vi "Modbus Slave Write Time.vi"() -> ()   [LabVIEW 2021]
doc: "An example of the modbus master functionality."
uses:
  Modbus_v121c/Network Protocol/Network Slave/daemon status.ctl
  Modbus_v121c/Network Protocol/Network Slave/TCP/Connection.ctl
  Modbus_v121c/Data Model/Identification Parameters.ctl
  Modbus_v121c/API/Slave/Modbus Slave.lvclass
  Modbus_v121c/Data Model/Device Data Model.lvclass
  Modbus_v121c/API/Wrapper/API Main.lvlib
  Modbus_v121c/Network Protocol/Network Slave/Network Slave.lvclass
  Modbus_v121c/Network Protocol/Network Slave/TCP/TCP Slave.lvclass
panel:
  out "TCP Connection List":T1[](array[typedef])=[{"Connected?"=TRUE, "IP address"="127.0.0.1", "connection error"={"status"=FALSE, "code"=0, "source"=""}}]
  out "TCP Connection Count":u32
  out "Daemon Error":errorcluster
  out "Daemon Status":T2
  in  "Port":u16=502
  in  "Basic Objects":string[](array[string])=["National Instruments", "42", "1.0.0"]
  out "Status":string
  out "Holding Registers":u16[](array[numeric])
  in  "Input Registers":u16[](array[numeric])=[0, 0, 0, 0, 0, 0, 0, 0]
  out "Coils":bool[](array[boolean])
  in  "Discrete Inputs":bool[](array[boolean])
  # "Holding Registers are the integer outputs of a modbus device. This example allows you to read the first 8 outputs."
  # "Coils are the boolean outputs of a modbus device. This example allows you to read the first 8 outputs."
  # "Modbus devices can also store objects in their memory, which are variable length strings. This example sets the basic level of objects."
  # "Discrete inputs are the boolean inputs of a modbus device. This example allows you to set the first 8 inputs."
  # "Input Registers are the integer inputs of a modbus device. This example allows you to set the first 8 inputs."
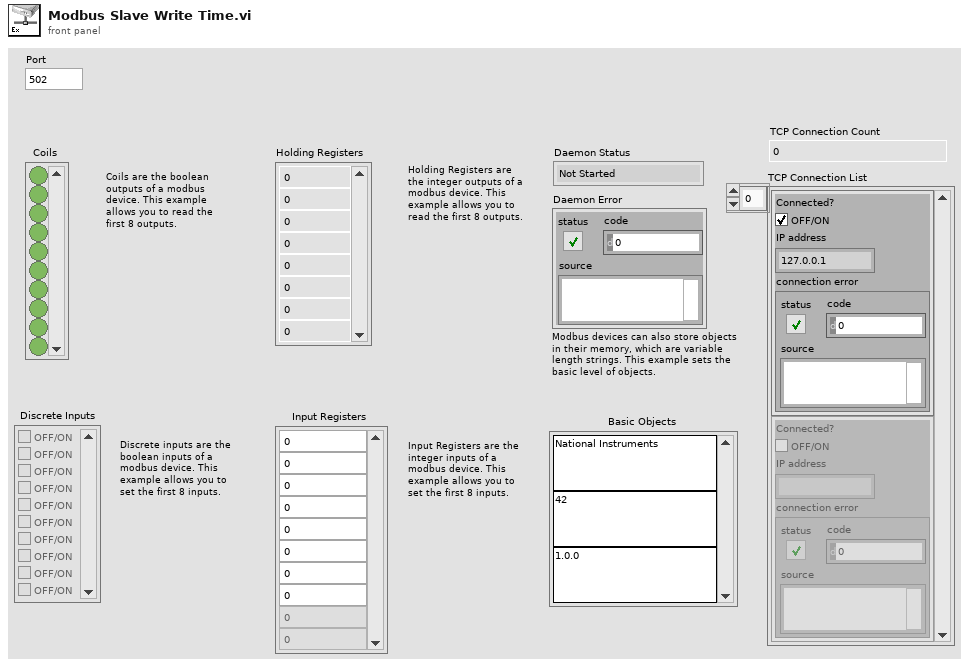
[diagram p1: front panel]
types:
  T1 = typedef "TCP Slave.lvclass/Connection.ctl" = cluster{"Connected?":bool, "IP address":string, "connection error":errorcluster}
  T2 = typedef "Network Slave.lvclass/daemon status.ctl" = enum16{"Not Started", "Running", "Error", "Stopped"}
  T3 = typedef "Device Data Model.lvclass/Identification Parameters.ctl" = cluster{"Object ID":u8, "Value":string}
  T4 = enum16{"Not Started", "Running", "Error", "Stopped"}
  T5 = cluster{"Connected?":bool, "IP address":string, "connection error":errorcluster}[]
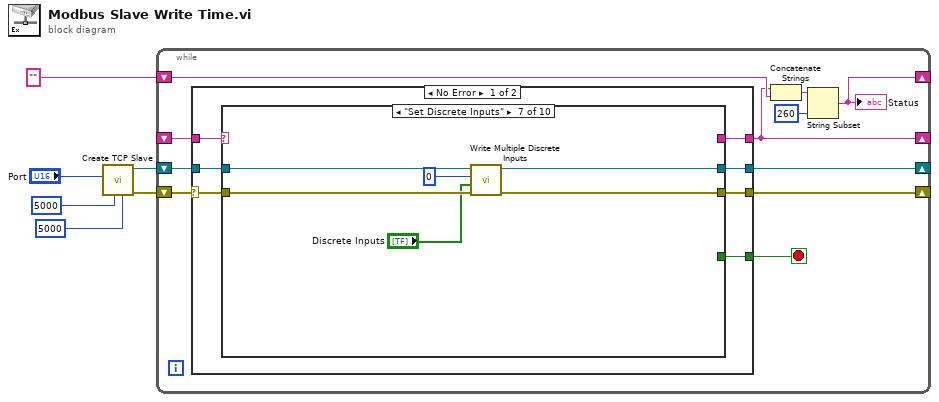
[diagram p0: block diagram]
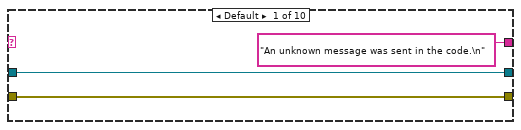
[diagram p2: hidden frame]
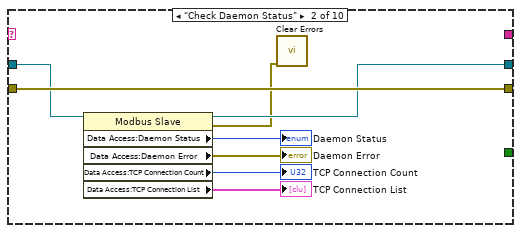
[diagram p3: hidden frame]
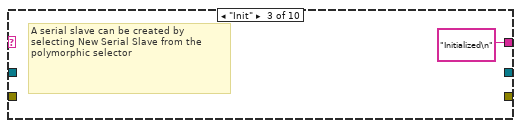
[diagram p4: hidden frame]
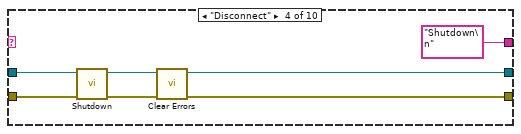
[diagram p5: hidden frame]
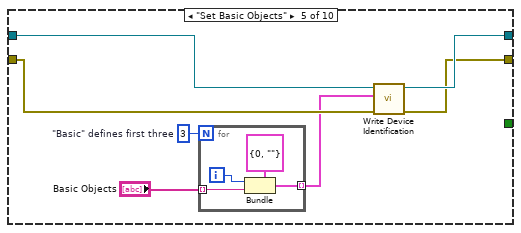
[diagram p6: hidden frame]
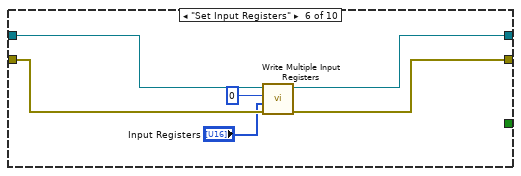
[diagram p7: hidden frame]
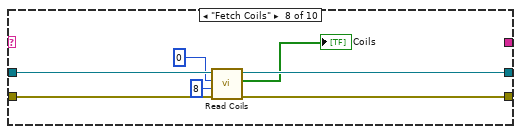
[diagram p8: hidden frame]
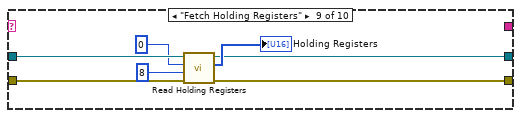
[diagram p9: hidden frame]
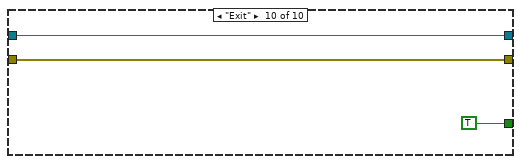
[diagram p10: hidden frame]
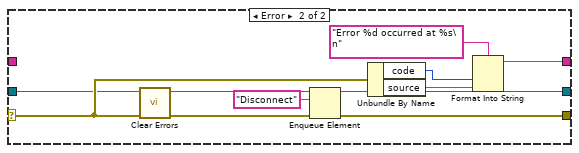
[diagram p11: hidden frame]
diagram:
  n1 = call "Create TCP Slave.vi"("write operation timeout"=5000, "read operation timeout"=5000, "port (502)"="Port") -> ("error out"=w3:errorcluster, "TCP slave instance"=w4:refnum<class "Modbus Slave.lvclass">)  [unwired: 7 in]
  n2 = while {
    shift-right: [w9] -> _
    shift-left: w4 -> [w12]
    shift-right: [w10] -> _
    shift-left: w3 -> [w17]
    shift-right: [w16] -> _
    shift-left: "" ("Status") -> [w13]
    shift-right: [w8] -> _
    shift-left: _ -> [w7]
    stop <- w11 stop-if-true
    n3 = case shown="No Error" w17 {
      selector: w17 -> [w19 w89]
      tunnel: [w24 w90] -> w10
      tunnel: [w21 w86] -> w8
      tunnel: [w23 w83] -> w9
      tunnel: w12 -> [w22 w83]
      tunnel: [w20 _] -> w11
      tunnel: w7 -> [w18 _]
      frame No Error {
        n4 = case shown="\"Set Discrete Inputs\"" w18 {
          tunnel: w19 -> [w27 w35 _ w42 w49 w56 w62 w69 w78 w82]
          tunnel: [w27 w35 _ w38 w44 w57 w63 w67 w75 w82] -> w24
          tunnel: [w26 w33 w37 w40 w48 w58 w64 w68 w76 w81] -> w23
          tunnel: w22 -> [w26 w34 _ w40 w47 w59 w65 w72 w79 w81]
          tunnel: ["An unknown message was sent in the code.\n" _ "Initialized\n" "Shutdown\n" _ _ _ _ _ _] -> w21
          tunnel: [_ _ _ _ _ _ _ _ _ TRUE] -> w20
          frame Default {
          }
          frame "Check Daemon Status" {
            n5 = property class="Modbus Slave"(reference=w34) -> (reference out=w33:refnum<class "Modbus Slave.lvclass">, error out=w32:errorcluster, "Data Access:Daemon Status"=→"Daemon Status":T4, "Data Access:Daemon Error"=→"Daemon Error":errorcluster, "Data Access:TCP Connection Count"=→"TCP Connection Count":u32, "Data Access:TCP Connection List"=→"TCP Connection List":T5)  [unwired: 1 in]
            n6 = call <vilib>:"Clear Errors.vi"("error in (no error)"=w32) -> ()  [unwired: 5 in, 2 out]
          }
          frame "Init" {
            # "A serial slave can be created by selecting New Serial Slave from the polymorphic selector"
          }
          frame "Disconnect" {
            n7 = call-dynamic "Shutdown.vi"("error in (no error)"=w42, "Modbus slave in"=w40) -> ("error out"=w41:errorcluster)  [unwired: 9 in]
            n8 = call <vilib>:"Clear Errors.vi"("error in (no error)"=w41) -> ("error out"=w38:errorcluster)  [unwired: 5 in, 1 out]
          }
          frame "Set Basic Objects" {
            w43 = 3  # "Basic" defines first three
            n9 = for {
              N: w43 -> [_]
              tunnel: "Basic Objects" -> [w51] mode=indexing
              tunnel: [w50] -> w45 mode=indexing
              i -> [w52]
              n10 = Bundle(cluster=T3 {"Object ID"=0, "Value"=""} ("Parameters"), "Object ID"=w52, "Value"=w51) -> (w50:T3)
            }
            n11 = call-dynamic "Write Device Identification.vi"("error in (no error)"=w49, "objects"=w45, "Modbus slave in"=w47) -> ("error out"=w44:errorcluster, "Modbus slave out"=w48:refnum<class "Modbus Slave.lvclass">)  [unwired: 7 in]
          }
          frame "Set Input Registers" {
            n12 = call-dynamic "Write Multiple Input Registers.vi"("error in (no error)"=w56, "input register values"="Input Registers", "starting address"=u16 0, "Modbus slave in"=w59) -> ("error out"=w57:errorcluster, "Modbus slave out"=w58:refnum<class "Modbus Slave.lvclass">)  [unwired: 6 in]
          }
          frame "Set Discrete Inputs" {
            n13 = call-dynamic "Write Multiple Discrete Inputs.vi"("error in (no error)"=w62, "discrete input values"="Discrete Inputs", "starting address"=u16 0, "Modbus slave in"=w65) -> ("error out"=w63:errorcluster, "Modbus slave out"=w64:refnum<class "Modbus Slave.lvclass">)  [unwired: 6 in]
          }
          frame "Fetch Coils" {
            n14 = call-dynamic "Read Coils.vi"("error in (no error)"=w69, "number of coils"=u16 8, "starting address"=u16 0, "Modbus slave in"=w72) -> ("error out"=w67:errorcluster, "coil values"=→"Coils":bool[], "Modbus slave out"=w68:refnum<class "Modbus Slave.lvclass">)  [unwired: 5 in]
          }
          frame "Fetch Holding Registers" {
            n15 = call-dynamic "Read Holding Registers.vi"("error in (no error)"=w78, "number of holding registers"=u16 8 ("number of registers"), "starting address"=u16 0, "Modbus slave in"=w79) -> ("error out"=w75:errorcluster, "register values"=→"Holding Registers":u16[], "Modbus slave out"=w76:refnum<class "Modbus Slave.lvclass">)  [unwired: 5 in]
          }
          frame "Exit" {
          }
        }
      }
      frame Error {
        n16 = call <vilib>:"Clear Errors.vi"("error in (no error)"=w89) -> ("error out"=w91:errorcluster)  [unwired: 5 in, 1 out]
        n17 = Enqueue Element(element="Disconnect", error in (no error)=w91) -> (error out=w90:errorcluster)  [unwired: 2 in, 2 out]
        n18 = Unbundle By Name(w89) -> ("code"=w88:i32, "source"=w87:string)
        n19 = Format Into String(format string="Error %d occurred at %s\n", w88, w87) -> (resulting string=w86:string)  [unwired: 2 in, 1 out]
      }
    }
    n20 = Concatenate Strings(w8, w13) -> (w14:string)
    n21 = String Subset(string=w14, length (rest)=260 ("length (rest)")) -> (substring=w16:string)  [unwired: 1 in]
    "Status" <- w16
  }
